vi "Read Action.vi"(8 "error in (no error)":errorcluster, 11 "AndrewF in":refnum<class "AndrewF.lvclass">) -> (0 "error out":errorcluster, 2 "Action":T1, 3 "AndrewF out":refnum<class "AndrewF.lvclass">)   [LabVIEW 2015, in "AndrewF.lvclass"]
uses:
  AndrewF.lvclass
  Type Defs/Action Enum.ctl
  AndrewF.lvclass/AndrewF.ctl
  Type Defs/SB Type Defs.lvlib
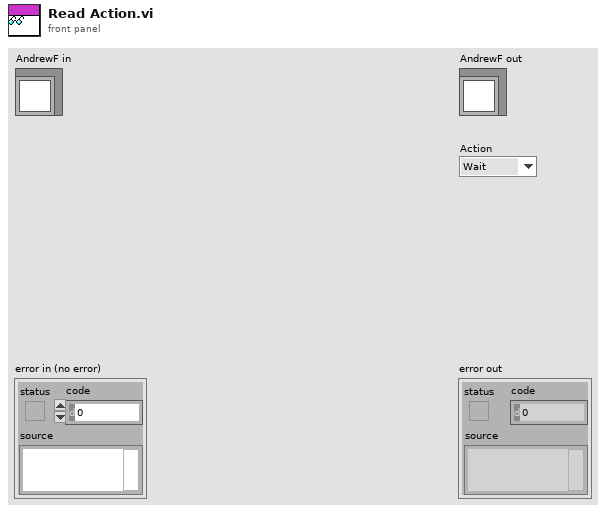
[diagram p1: front panel]
types:
  T1 = typedef "SB Type Defs.lvlib/Action Enum.ctl" = enum16{"Wait", "Move", "Attack", "Replicate"}
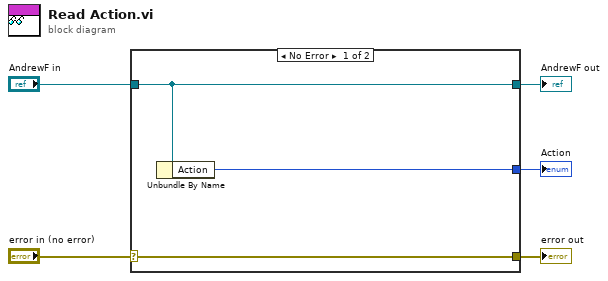
[diagram p0: block diagram]
diagram:
  n1 = case shown="No Error" "error in (no error)" {
    selector: "error in (no error)" -> [w8 w9]
    tunnel: [w8 w9] -> w4
    tunnel: [w7 w10] -> w2
    tunnel: "AndrewF in" -> [w7 w10]
    tunnel: [w6 _] -> w1
    frame No Error {
      n2 = Unbundle By Name(w7) -> ("Action"=w6:T1)
    }
    frame Error {
    }
  }
  "error out" <- w4
  "AndrewF out" <- w2
  "Action" <- w1
